vi "Demo - Transient Capture (Multiple Shots).vi"(6 "Soft Trigger":bool=TRUE, 9 "Post-Trigger Samples":i32=100000, 10 "Pre-Trigger Samples":i32, 11 "configuration file path":path) -> ()   [LabVIEW 2017]
doc: "Demonstration of transient capture mode, in a continuos loop"
uses:
  Communications/Communications Library.lvlib
  GUI/Consoles/Communications Console Library.lvlib
panel:
  in  "Show Console":bool
  in  "stop":bool
  in  "ARM":bool
  out "Waveform Graph":i16[][](graph)
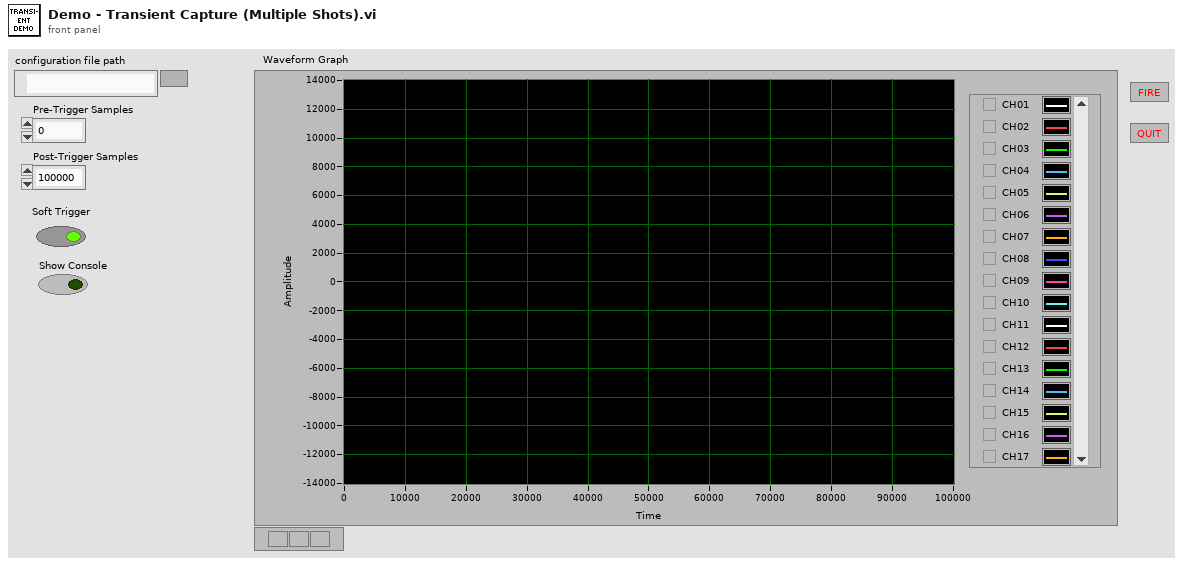
[diagram p1: front panel]
types:
  T1 = typedef "Communications Library.lvlib/DTACQ Module Carrier Configuration--Cluster.ctl" = cluster{"Name":string, "IP":string, "Control Port":i32, "Timeout (ms)":i32, "Continuous Capture Port (Multiplexed)":i32, "Start HIL Shot Port":i32, "AWG Upload Port (Multiplexed)":i32, "Download Captured Data Port (Multiplexed)":i32, "Module Slots":i32, "Module Configurations":T2[]}
  T2 = typedef "Communications Library.lvlib/DTACQ Module Configuration--Cluster.ctl" = cluster{"Name":string, "Position":string, "Module Type":T3, "Control Port":i32, "Timeout (ms)":i32, "Channels":i32}
  T3 = typedef "Communications Library.lvlib/DTACQ Device Type--Enum.ctl" = enum16{"Carrier", "Analog In Module", "Analog Out Module", "Generic Module"}
  T4 = typedef "Communications Library.lvlib/DTACQ Connection Data--Cluster.ctl" = cluster{"Description":string, "Address":string, "Port":u16, "timeout (ms)":i32, "Termination Character":string, "TCP Connection Reference":refnum<k5>, "Open Connection":bool}
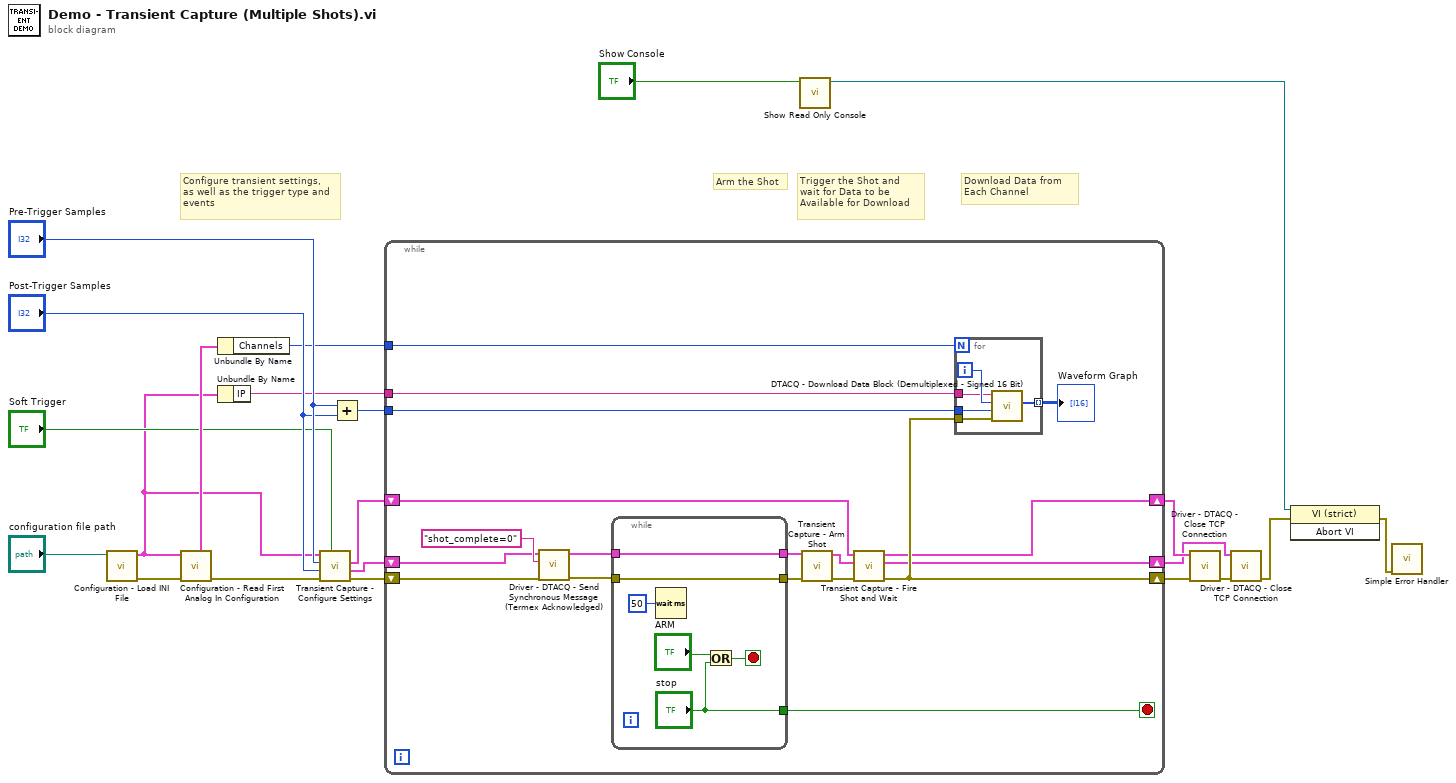
[diagram p0: block diagram]
diagram:
  # "Configure transient settings,\nas well as the trigger type and\nevents"
  # "Trigger the Shot and\nwait for Data to be\nAvailable for Download"
  # "Download Data from \nEach Channel"
  # "Arm the Shot"
  n1 = call "Configuration - Load INI File.vi"("configuration file path"="configuration file path") -> ("error out"=w18:errorcluster, "Carrier Configuration Out"=w1:T1)  [unwired: 9 in]
  n2 = call "Configuration - Read First Analog In Configuration.vi"("error in"=w18, "Carrier Configuration"=w1) -> ("error out"=w17:errorcluster, "AI - Module Configuration"=w19:T2)  [unwired: 5 in, 3 out]
  n3 = Unbundle By Name(w19) -> ("Channels"=w8:i32)
  n4 = Unbundle By Name(w1) -> ("IP"=w14:string)
  n5 = call "Transient Capture - Configure Settings.vi"("Soft Trigger"="Soft Trigger", "error in"=w17, "Samples to Read (Post Trigger)"="Post-Trigger Samples", "Samples to Read (Pre Trigger)"="Pre-Trigger Samples", "Carrier Configuration"=w1) -> ("error out"=w15:errorcluster, "Carrier Connection Out"=w7:T4, "AI Connection Out"=w6:T4)  [unwired: 4 in]
  n6 = Add(x="Pre-Trigger Samples", y="Post-Trigger Samples") -> (x+y=w13:i32)
  n7 = while {
    tunnel: w14 -> [w37]
    tunnel: w13 -> [w36]
    tunnel: w8 -> [w32]
    shift-right: [w35] -> w12
    shift-left: w15 -> [w26]
    shift-right: [w34] -> w10
    shift-left: w6 -> [w29]
    shift-right: [w33] -> w9
    shift-left: w7 -> [w25]
    stop <- w28 stop-if-true
    n8 = call "Driver - DTACQ - Send Synchronous Message (Termex Acknowledged).vi"("error in"=w26, "Message to Send"="shot_complete=0", "DTACQ Connection Data In"=w25) -> ("error out"=w23:errorcluster, "DTACQ Connection Data Out"=w24:T4)  [unwired: 5 in, 2 out]
    n9 = while {
      tunnel: [w41] -> w39
      tunnel: [w42] -> w31
      tunnel: ["stop"] -> w28
      tunnel: w24 -> [w42]
      tunnel: w23 -> [w41]
      stop <- w43 stop-if-true
      n10 = Wait (ms)(milliseconds to wait=u32 50) -> ()  [unwired: 1 out]
      n11 = Or(x="ARM", y="stop") -> (x .or. y?=w43:bool)
    }
    n12 = call "Transient Capture - Arm Shot.vi"("error in"=w39, "Carrier Connection In"=w31) -> ("error out"=w38:errorcluster, "DTACQ Connection Out"=w30:T4)  [unwired: 8 in]
    n13 = call "Transient Capture - Fire Shot and Wait.vi"("error in"=w38, "Carrier Connection In"=w30, "AI Connection In"=w29) -> ("error out"=w35:errorcluster, "Carrier Connection Out"=w33:T4, "AI Connection Out"=w34:T4)  [unwired: 6 in]
    n14 = for {
      N: w32 -> [_]
      tunnel: [w50] -> w40 mode=indexing
      tunnel: w36 -> [w49]
      tunnel: w37 -> [w48]
      tunnel: w35 -> [w47]
      i -> [w51]
      n15 = call "DTACQ - Download Data Block (Demultiplexed - Signed 16 Bit).vi"("error in"=w47, "Maximum Number of Samples"=w49, "Channel Number"=w51, "Address"=w48) -> ("(Signed) 16 Bit Array"=w50:i16[])  [unwired: 5 in, 2 out]
    }
    "Waveform Graph" <- w40
  }
  n16 = call "Show Read Only Console.vi"("Show Console"="Show Console") -> ("VI out"=w4:refnum<vi>)  [unwired: 10 in]
  n17 = call "Driver - DTACQ - Close TCP Connection.vi"("error in"=w12, "DTACQ Connection Data In"=w10) -> ("error out"=w11:errorcluster)  [unwired: 8 in, 1 out]
  n18 = call "Driver - DTACQ - Close TCP Connection.vi"("error in"=w11, "DTACQ Connection Data In"=w9) -> ("error out"=w3:errorcluster)  [unwired: 8 in, 1 out]
  n19 = invoke class="VI (strict)" method="Abort VI"(reference=w4, error in=w3) -> (error out=w2:errorcluster)  [unwired: 1 in, 2 out]
  n20 = call <vilib>:"Simple Error Handler.vi"("error in (no error)"=w2) -> ()  [unwired: 4 in, 5 out]
